vi "RotationGlobal.vi"() -> ()   [LabVIEW 2012]
uses:
  Event/MainEvents.ctl
panel:
  in  "Path of CalCurve File":path
  in  "Step Size (deg)":dbl=1.0
  in  "Final Angle (deg)":dbl=45.0
  in  "Initial Angle (deg)":dbl
  in  "theta opt":dbl
  in  "formula Cal Curve":string
  in  "Stage Sync Data File":path
  in  "formula":string
  in  "theta0":dbl
  out "Current Angle (deg)":dbl=1.4990625
  in  "Move Abs (deg)":dbl=25.0
  out "Rotation events":refnum<queue>
  # "Surf Cal V2"
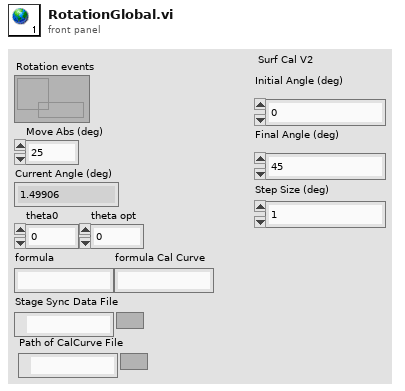
[diagram p1: front panel]
diagram:
